vi "总磷氨氮测量数据储存.vi"   [LabVIEW 2016, in "斯坦道仪器.lvlib"]
types:
  T1 = cluster{"时间标识":timestamp, "监测值":sgl, "单位":u16, "数据标识":string, "因子编码":u32, "标样参考值":sgl, "F0":sgl, "F1":sgl, "F2":sgl, "F3":sgl, "F4":sgl, "F5":sgl, "F6":sgl, "F7":sgl, "X":sgl, "温度":sgl, "湿度":sgl, "量程标识":string}
  T2 = enum16{"维护数据", "水样测试", "标样核查", "零点核查", "跨度核查", "空白测试", "平行样测试", "加标回收", "空白校准", "标样校准", "初始化（清洗）"}
  T3 = cluster{"系统时间":timestamp, "工作状态":enum16{"空闲", "水样测试", "标样核查", "零点核查", "跨度核查", "空白测试", "平行样测试", "加标回收", "空白校准", "标样校准", "初始化（清洗）"}, "测量模式":enum16{"待机", "连续模式", "周期模式", "定点模式", "受控模式", "手动模式"}, "告警代码":enum16{"无告警", "缺试剂告警", "缺水样告警", "缺蒸馏水告警", "缺标液告警", "仪表漏液告警", "标定异常告警", "超量程告警", "加热异常", "低试剂预警", "超上限告警", "超下限告警", "仪表内部其他异常", "滴定异常告警", "电极异常告警", "量程切换告警", "参数设置告警", "PH电极电位异常", "电导率电极异常", "浊度光度异常", "溶解氧电极异常", "溶解氧光强异常", "温度异常告警", "PH异常告警", "溶解氧异常告警", "电导率异常告警", "浊度异常告警", "叶绿素异常告警", "藻密度异常告警", "蓝绿藻异常告警", "ORP异常告警", "氨氮异常告警", "清洁刷异常告警", "SD卡异常告警", "蓝牙异常告警", "Wifi异常告警", "流程异常告警"}, "故障代码":enum16{"无故障", "电机故障", "温度故障", "通讯故障", "滴定故障"}, "日志代码":u16, "软件版本":u16, "F0":sgl, "F1":sgl, "F2":sgl, "F3":sgl, "T":sgl, "H":sgl, "id":u16, "flowid":u16, "量程":u16}
  T4 = enum16{"空闲", "水样测试", "标样核查", "零点核查", "跨度核查", "空白测试", "平行样测试", "加标回收", "空白校准", "标样校准", "初始化（清洗）"}
  T5 = cluster{"因子编码":u32, "单位":u16, "标样参考值":sgl, "水样数据时间":timestamp, "水样实测值":sgl, "水样数据标识":string, "标样数据时间":timestamp, "标样实测值":sgl, "标样数据标识":string, "空白数据时间":timestamp, "空白实测值":sgl, "空白数据标识":string, "零点核查数据时间":timestamp, "零点核查实测值":sgl, "零点核查数据标识":string, "跨度核查数据时间":timestamp, "跨度核查实测值":sgl, "跨度核查数据标识":string, "加标回收数据时间":timestamp, "加标回收实测值":sgl, "加标回收数据标识":string, "平行样数据时间":timestamp, "平行样实测值":sgl, "平行样数据标识":string, "F0":sgl, "F1":sgl, "F2":sgl, "F3":sgl, "F4":sgl, "F5":sgl, "F6":sgl, "F7":sgl, "温度":sgl, "湿度":sgl, "X值":sgl}
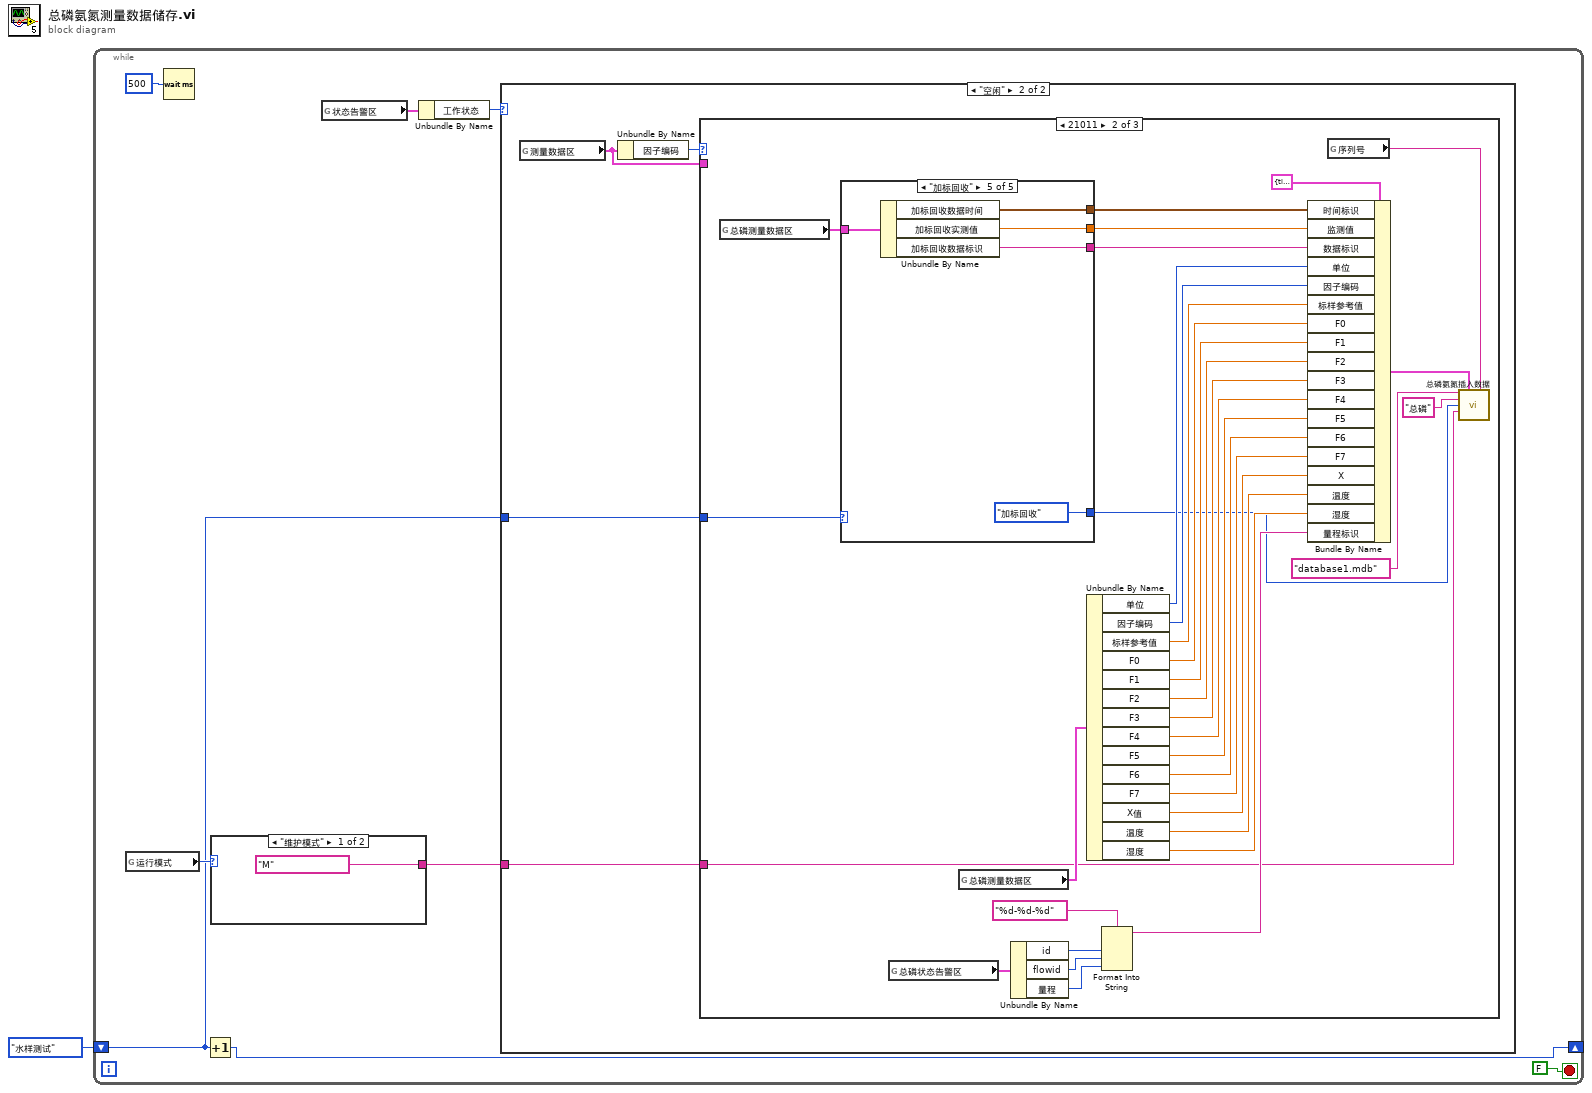
[diagram p0: block diagram]
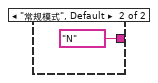
[diagram p2: hidden frame]
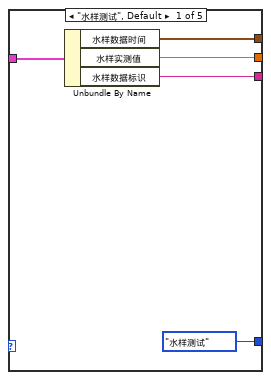
[diagram p5: hidden frame]
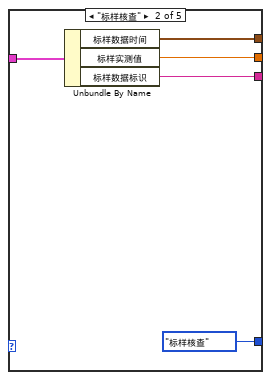
[diagram p6: hidden frame]
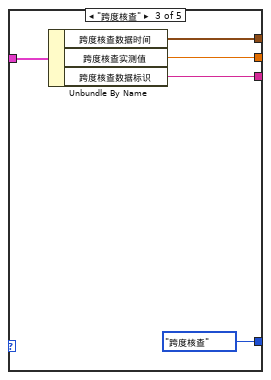
[diagram p7: hidden frame]
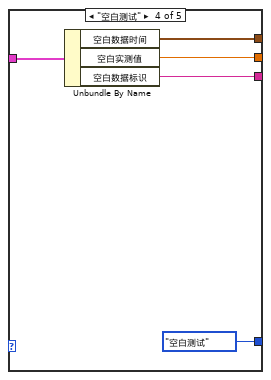
[diagram p8: hidden frame]
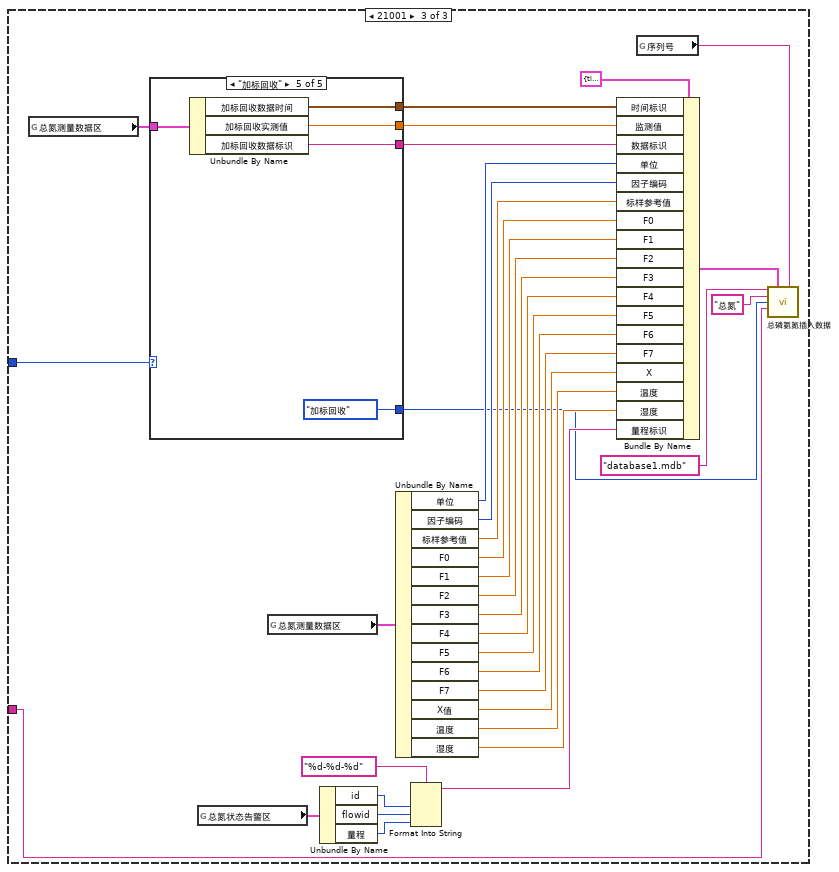
[diagram p9: hidden frame]
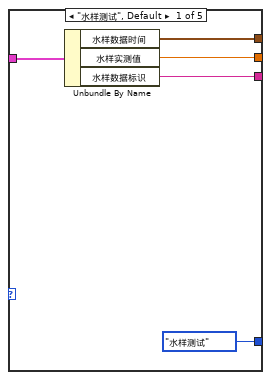
[diagram p10: hidden frame]
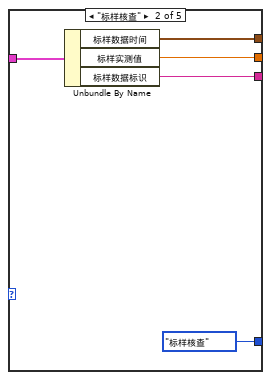
[diagram p11: hidden frame]
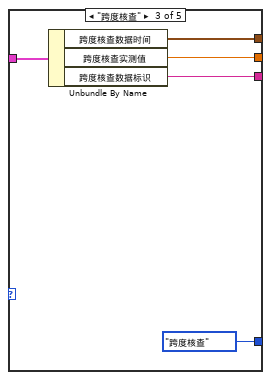
[diagram p12: hidden frame]
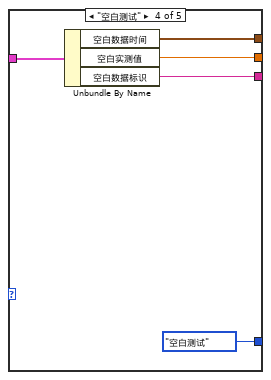
[diagram p13: hidden frame]
diagram:
  n1 = while {
    shift-right: [w4] -> _
    shift-left: enum16{"水样测试", "标样核查", "跨度核查", "空白测试", "加标回收"}."水样测试" ("测量模式") -> [w3]
    stop <- FALSE stop-if-true
    n2 = global read "系统变量.vi" "运行模式"() -> (w6:enum16{"维护模式", "常规模式", "应急模式", "质控模式"})
    n3 = Wait (ms)(milliseconds to wait=u32 500 ("等待时间（毫秒）")) -> ()  [unwired: 1 out]
    n4 = Increment(x=w3) -> (x+1=w4:enum16{"水样测试", "标样核查", "跨度核查", "空白测试", "加标回收"})
    n5 = case shown="\"维护模式\"" w6 {
      tunnel: ["M" ("数据标记表") "N" ("数据标记表")] -> w5
      frame "维护模式" {
      }
      frame "常规模式", Default {
      }
    }
    n6 = global read "VAR总磷氨氮全局变量.vi" "状态告警区"() -> (w2:T3)
    n7 = Unbundle By Name(w2) -> ("工作状态"=w7:T4)
    n8 = case shown="\"空闲\"" w7 {
      tunnel: w5 -> [_ w13]
      tunnel: w3 -> [_ w12]
      frame Default {
      }
      frame "空闲" {
        n9 = global read "VAR总磷氨氮全局变量.vi" "测量数据区"() -> (w15:T5)
        n10 = Unbundle By Name(w15) -> ("因子编码"=w14:u32)
        n11 = case shown="21011" w14 {
          tunnel: w15 -> [_ _ _]
          tunnel: w13 -> [_ w18 w94]
          tunnel: w12 -> [_ w17 w79]
          frame Default {
          }
          frame 21011 {
            n12 = global read "VAR总磷氨氮全局变量.vi" "总磷测量数据区"() -> (w47:T5)
            n13 = case shown="\"加标回收\"" w17 {
              tunnel: w47 -> [w53 w58 w63 w68 w73]
              tunnel: [w52 w57 w62 w67 w72] -> w22
              tunnel: [w51 w56 w61 w66 w71] -> w23
              tunnel: [w50 w55 w60 w65 w70] -> w24
              tunnel: [T2."水样测试" ("测量模式") T2."标样核查" ("测量模式") T2."跨度核查" ("测量模式") T2."空白测试" ("测量模式") T2."加标回收" ("测量模式")] -> w21
              frame "水样测试", Default {
                n14 = Unbundle By Name(w53) -> ("水样数据时间"=w52:timestamp, "水样实测值"=w51:sgl, "水样数据标识"=w50:string)
              }
              frame "标样核查" {
                n15 = Unbundle By Name(w58) -> ("标样数据时间"=w57:timestamp, "标样实测值"=w56:sgl, "标样数据标识"=w55:string)
              }
              frame "跨度核查" {
                n16 = Unbundle By Name(w63) -> ("跨度核查数据时间"=w62:timestamp, "跨度核查实测值"=w61:sgl, "跨度核查数据标识"=w60:string)
              }
              frame "空白测试" {
                n17 = Unbundle By Name(w68) -> ("空白数据时间"=w67:timestamp, "空白实测值"=w66:sgl, "空白数据标识"=w65:string)
              }
              frame "加标回收" {
                n18 = Unbundle By Name(w73) -> ("加标回收数据时间"=w72:timestamp, "加标回收实测值"=w71:sgl, "加标回收数据标识"=w70:string)
              }
            }
            n19 = global read "VAR总磷氨氮全局变量.vi" "总磷状态告警区"() -> (w16:T3)
            n20 = global read "VAR总磷氨氮全局变量.vi" "总磷测量数据区"() -> (w29:T5)
            n21 = Unbundle By Name(w16) -> ("id"=w48:u16, "flowid"=w31:u16, "量程"=w30:u16)
            n22 = Unbundle By Name(w29) -> ("单位"=w46:u16, "因子编码"=w45:u32, "标样参考值"=w44:sgl, "F0"=w43:sgl, "F1"=w42:sgl, "F2"=w41:sgl, "F3"=w40:sgl, "F4"=w39:sgl, "F5"=w38:sgl, "F6"=w37:sgl, "F7"=w36:sgl, "X值"=w35:sgl, "温度"=w34:sgl, "湿度"=w33:sgl)
            n23 = Format Into String(format string="%d-%d-%d" ("格式字符串"), w48, w31, w30) -> (resulting string=w32:string)  [unwired: 2 in, 1 out]
            n24 = Bundle By Name(cluster=T1 {"时间标识"=timestamp(0 s since 1904-01-01), "监测值"=0.0, "单位"=0, "数据标识"="", "因子编码"=0, "标样参考值"=0.0, "F0"=0.0, "F1"=0.0, "F2"=0.0, "F3"=0.0, "F4"=0.0, "F5"=0.0, "F6"=0.0, "F7"=0.0, "X"=0.0, "温度"=0.0, "湿度"=0.0, "量程标识"=""} ("data"), "时间标识"=w22, "监测值"=w23, "数据标识"=w24, "单位"=w46, "因子编码"=w45, "标样参考值"=w44, "F0"=w43, "F1"=w42, "F2"=w41, "F3"=w40, "F4"=w39, "F5"=w38, "F6"=w37, "F7"=w36, "X"=w35, "温度"=w34, "湿度"=w33, "量程标识"=w32) -> (w26:T1)
            n25 = global read "VAR总磷氨氮全局变量.vi" "序列号"() -> (w25:string)
            n26 = call "总磷氨氮插入数据.vi"("database"="database1.mdb", "data"=w26, "SN"=w25, "table"="总磷", "测量模式"=w21, "数据标记表"=w18) -> ()  [unwired: 9 in, 1 out]
          }
          frame 21001 {
            n27 = global read "VAR总磷氨氮全局变量.vi" "总氮测量数据区"() -> (w78:T5)
            n28 = case shown="\"加标回收\"" w79 {
              tunnel: w78 -> [w111 w116 w121 w126 w131]
              tunnel: [w110 w115 w120 w125 w130] -> w77
              tunnel: [w109 w114 w119 w124 w129] -> w76
              tunnel: [w108 w113 w118 w123 w128] -> w75
              tunnel: [T2."水样测试" ("测量模式") T2."标样核查" ("测量模式") T2."跨度核查" ("测量模式") T2."空白测试" ("测量模式") T2."加标回收" ("测量模式")] -> w74
              frame "水样测试", Default {
                n29 = Unbundle By Name(w111) -> ("水样数据时间"=w110:timestamp, "水样实测值"=w109:sgl, "水样数据标识"=w108:string)
              }
              frame "标样核查" {
                n30 = Unbundle By Name(w116) -> ("标样数据时间"=w115:timestamp, "标样实测值"=w114:sgl, "标样数据标识"=w113:string)
              }
              frame "跨度核查" {
                n31 = Unbundle By Name(w121) -> ("跨度核查数据时间"=w120:timestamp, "跨度核查实测值"=w119:sgl, "跨度核查数据标识"=w118:string)
              }
              frame "空白测试" {
                n32 = Unbundle By Name(w126) -> ("空白数据时间"=w125:timestamp, "空白实测值"=w124:sgl, "空白数据标识"=w123:string)
              }
              frame "加标回收" {
                n33 = Unbundle By Name(w131) -> ("加标回收数据时间"=w130:timestamp, "加标回收实测值"=w129:sgl, "加标回收数据标识"=w128:string)
              }
            }
            n34 = global read "VAR总磷氨氮全局变量.vi" "总氮状态告警区"() -> (w102:T3)
            n35 = global read "VAR总磷氨氮全局变量.vi" "总氮测量数据区"() -> (w106:T5)
            n36 = Unbundle By Name(w102) -> ("id"=w98:u16, "flowid"=w97:u16, "量程"=w96:u16)
            n37 = Unbundle By Name(w106) -> ("单位"=w105:u16, "因子编码"=w104:u32, "标样参考值"=w103:sgl, "F0"=w92:sgl, "F1"=w91:sgl, "F2"=w90:sgl, "F3"=w89:sgl, "F4"=w88:sgl, "F5"=w87:sgl, "F6"=w86:sgl, "F7"=w85:sgl, "X值"=w84:sgl, "温度"=w83:sgl, "湿度"=w82:sgl)
            n38 = Format Into String(format string="%d-%d-%d" ("格式字符串"), w98, w97, w96) -> (resulting string=w81:string)  [unwired: 2 in, 1 out]
            n39 = Bundle By Name(cluster=T1 {"时间标识"=timestamp(0 s since 1904-01-01), "监测值"=0.0, "单位"=0, "数据标识"="", "因子编码"=0, "标样参考值"=0.0, "F0"=0.0, "F1"=0.0, "F2"=0.0, "F3"=0.0, "F4"=0.0, "F5"=0.0, "F6"=0.0, "F7"=0.0, "X"=0.0, "温度"=0.0, "湿度"=0.0, "量程标识"=""} ("data"), "时间标识"=w77, "监测值"=w76, "数据标识"=w75, "单位"=w105, "因子编码"=w104, "标样参考值"=w103, "F0"=w92, "F1"=w91, "F2"=w90, "F3"=w89, "F4"=w88, "F5"=w87, "F6"=w86, "F7"=w85, "X"=w84, "温度"=w83, "湿度"=w82, "量程标识"=w81) -> (w80:T1)
            n40 = global read "VAR总磷氨氮全局变量.vi" "序列号"() -> (w95:string)
            n41 = call "总磷氨氮插入数据.vi"("database"="database1.mdb", "data"=w80, "SN"=w95, "table"="总氮", "测量模式"=w74, "数据标记表"=w94) -> ()  [unwired: 9 in, 1 out]
          }
        }
      }
    }
  }
